vi "Experimental vision.vi"() -> ()   [LabVIEW 2018]
uses:
  <vilib>/vision/driver/NI_Vision_Acquisition_Software.lvlib
  <vilib>/userdefined/High Color/IMAQdx.ctl
panel:
  out "Image Out 2":T1(plugin-control)
  in  "stop":bool
  out "error out":errorcluster
  out "Image Out":T1(plugin-control)
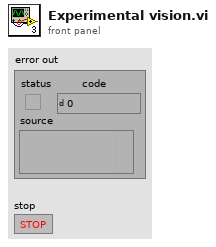
[diagram p1: front panel]
types:
  T1 = typedef "IMAQ Image.ctl" = refnum<image>
  T2 = typedef "IMAQdx.ctl" = refnum<k21>
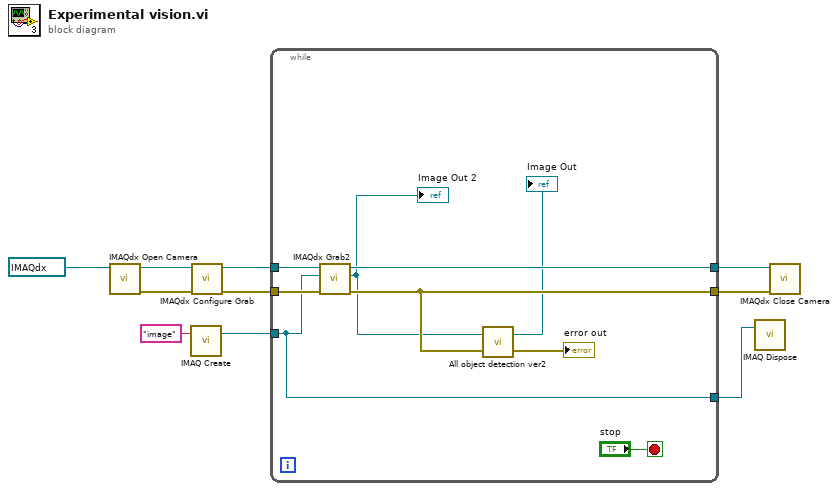
[diagram p0: block diagram]
diagram:
  n1 = call <vilib>:"IMAQdx Open Camera.vi"("Session In"=T2 "cam1") -> ("error out"=w7:errorcluster, "Session Out"=w10:T2)  [unwired: 9 in]
  n2 = call "IMAQ Create"("Image Name"="image") -> ("New Image"=w4:T1)  [unwired: 4 in, 1 out]
  n3 = call <vilib>:"IMAQdx Configure Grab.vi"("error in"=w7, "Session In"=w10) -> ("error out"=w6:errorcluster, "Session Out"=w9:T2)  [unwired: 8 in]
  n4 = while {
    tunnel: w9 -> [w19]
    tunnel: [w18] -> w8
    tunnel: w6 -> [w17]
    tunnel: [w16] -> w5
    tunnel: w4 -> [w12]
    tunnel: [w12] -> w2
    stop <- "stop" stop-if-true
    n5 = call <vilib>:"IMAQdx Grab2.vi"("error in"=w17, "Image In"=w12, "Session In"=w19) -> ("error out"=w16:errorcluster, "Image Out"=w11:T1, "Session Out"=w18:T2)  [unwired: 5 in, 1 out]
    "Image Out 2" <- w11
    n6 = call "All object detection ver2.vi"("error in"=w16, "Image In"=w11) -> ("error out"=→"error out":errorcluster, "Image Out"=→"Image Out":T1)
  }
  n7 = call "IMAQ Dispose"("Image"=w2) -> ()  [unwired: 5 in, 1 out]
  n8 = call <vilib>:"IMAQdx Close Camera.vi"("error in"=w5, "Session In"=w8) -> ()  [unwired: 9 in, 1 out]
